vi "Set Color Alpha.vi"(1 "Alpha":u8, 2 "Color In":u32(colorbox)) -> (0 "Color Out":u32(colorbox))   [LabVIEW 2023, in "Glyph Drawer.lvlib"]
uses:
  Glyph/Glyph Drawer.lvlib
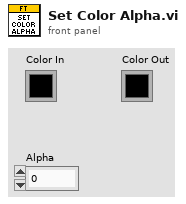
[diagram p1: front panel]
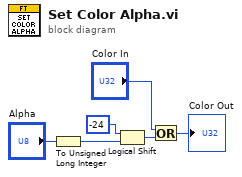
[diagram p0: block diagram]
diagram:
  n1 = To Unsigned Long Integer(number="Alpha") -> (unsigned 32bit integer=w3:u32)
  n2 = Logical Shift(y=i16 -24, x=w3) -> (x << y=w2:u32)
  n3 = Or(x="Color In", y=w2) -> (x .or. y?=→"Color Out":u32)
